vi "GetCaseNames.vi"(7 "ClassName":string, 8 "error in (no error)":errorcluster, 9 "DiagramIndex":i32, 10 "DiagramCount":i32, 11 "MultiFrameStructure in":refnum<vi>) -> (0 "error out":errorcluster, 2 "String":string, 3 "MultiFrameStructure out":refnum<vi>)   [LabVIEW 2017]
doc: "Returns Pattern name for the case"
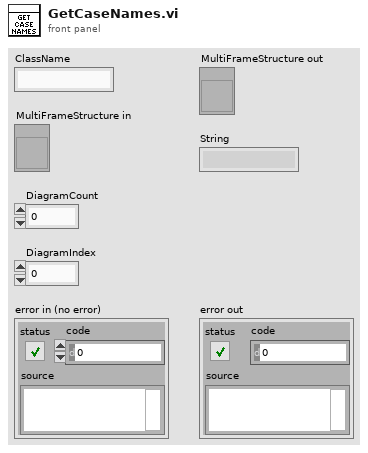
[diagram p1: front panel]
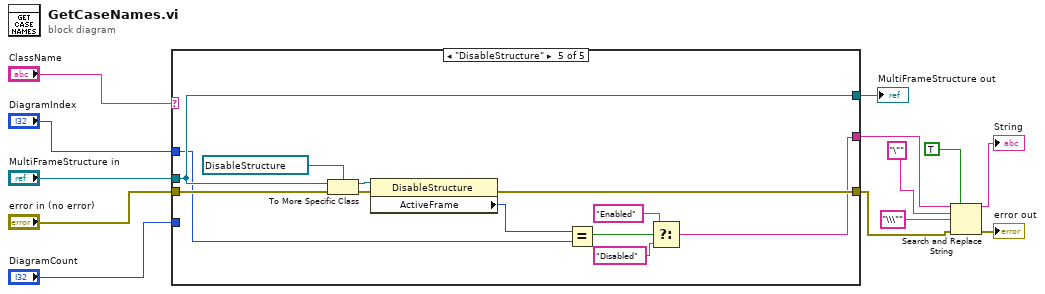
[diagram p0: block diagram]
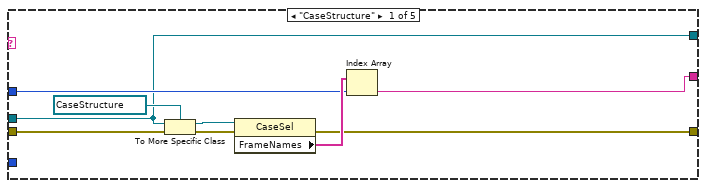
[diagram p2: hidden frame]
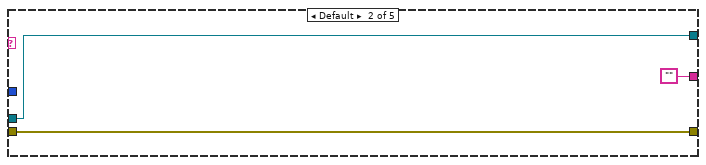
[diagram p3: hidden frame]
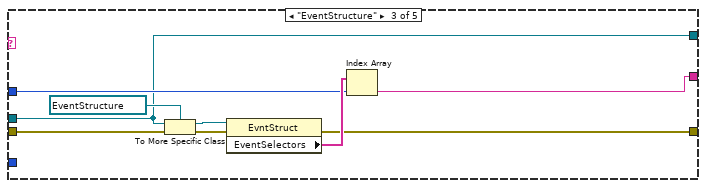
[diagram p4: hidden frame]
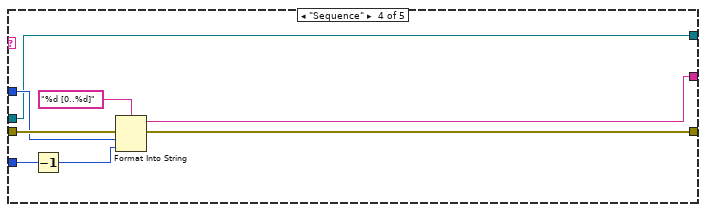
[diagram p5: hidden frame]
diagram:
  n1 = case shown="\"DisableStructure\"" "ClassName" {
    tunnel: "MultiFrameStructure in" -> [w14 w23 w26 w35 w51]
    tunnel: "error in (no error)" -> [w22 w24 w34 w41 w54]
    tunnel: "DiagramIndex" -> [w17 _ w29 w38 w46]
    tunnel: [w16 "" w28 w39 w47] -> w7
    tunnel: [w15 w24 w27 w40 w50] -> w4
    tunnel: "DiagramCount" -> [_ _ _ w37 _]
    tunnel: [w14 w23 w26 w35 w51] -> w13
    frame "CaseStructure" {
      n2 = To More Specific Class(target class=refnum<vi> refnum ("specific class reference"), reference=w14, error in=w22) -> (specific class reference=w20:refnum<vi>, error out=w21:errorcluster)
      n3 = property class="CaseSel"(reference=w20, error in=w21) -> (error out=w15:errorcluster, "FrameNames"=w18:string[])  [unwired: 1 out]
      n4 = Index Array(array=w18, index=w17) -> (element=w16:string)
    }
    frame Default {
    }
    frame "EventStructure" {
      n5 = To More Specific Class(target class=refnum<vi> refnum ("specific class reference"), reference=w26, error in=w34) -> (specific class reference=w32:refnum<vi>, error out=w33:errorcluster)
      n6 = property class="EvntStruct"(reference=w32, error in=w33) -> (error out=w27:errorcluster, "EventSelectors"=w30:string[])  [unwired: 1 out]
      n7 = Index Array(array=w30, index=w29) -> (element=w28:string)
    }
    frame "Sequence" {
      n8 = Decrement(x=w37) -> (x-1=w36:i32)
      n9 = Format Into String(format string="%d [0..%d]", error in=w41, w38, w36) -> (resulting string=w39:string, error out=w40:errorcluster)  [unwired: 1 in]
    }
    frame "DisableStructure" {
      n10 = To More Specific Class(target class=refnum<vi> refnum ("specific class reference"), reference=w51, error in=w54) -> (specific class reference=w49:refnum<vi>, error out=w53:errorcluster)
      n11 = property class="DisableStructure"(reference=w49, error in=w53) -> (error out=w50:errorcluster, "ActiveFrame"=w48:i16)  [unwired: 1 out]
      n12 = Equal?(x=w48, y=w46) -> (x = y?=w45:bool)
      n13 = Select(t="Enabled", s=w45, f="Disabled") -> (s? t:f=w47:string)
    }
  }
  "MultiFrameStructure out" <- w13
  n14 = Search and Replace String(replace all?=TRUE ("replace all? (F)"), input string=w7, search string="\"", replace string="\\\"" ("replace string (\"\")"), error in=w4) -> (result string=→"String":string, error out=→"error out":errorcluster)  [unwired: 3 in, 2 out]
